vi "Calc Calculated Values 2.vi"(8 "error in":errorcluster, 10 "RT - Analysis Data in":T4={"Accel Sensistivity"=[0.0, 0.0, 0.0], "Cutoff Frequncies"=[{"LP Passband"=0.0, "HP Stopband"=0.0, "LP Stopband"=0.0, "HP Passband"=0.0}, {"LP Passband"=0.0, "HP Stopband"=0.0, "LP Stopband"=0.0, "HP Passband"=0.0}, {"LP Passband"=0.0, "HP Stopband"=0.0, "LP Stopband"=0.0, "HP Passband"=0.0}], "APU Setup File"={"Sensor Info"=[], "CMM Table 106"=[], "CMM Table 106B "=[], "Accel Config"=[], "Report Sheet 1"=[], "Report Sheet 2"=[], "Report Sheet 3"=[]}, "RepairLevel"=""} {"Cutoff Frequncies"."HP Passband" min=1.0 step=1.0 format="%#.4f"; "Cutoff Frequncies"."LP Stopband" min=1.0 step=1.0 format="%#.4f"; "Cutoff Frequncies"."HP Stopband" min=1.0 step=1.0 format="%#.4f"; "Cutoff Frequncies"."LP Passband" min=1.0 step=1.0 format="%#.4f"}, 11 "All Data":T1 caption="All Data Cluster") -> (0 "error out":errorcluster, 3 "Calculated Values out":T3)   [LabVIEW 2018, in "RT - Analysis.lvlib"]
doc: "Performs all calculations to get the calculated values. Default output for a calculated value without an assigned calculation is NaN."
uses:
  RT - Analysis.lvlib
  Top Level/Shared Controls/Calculated Data.ctl
  <userlib>/_OpenG.lib/array/array.llb/Reorder 1D Array2 (DBL)__ogtk.vi
  Private Controls/RT-Analysis Data.ctl
  Modules/Testing UI 3/Private Controls/Cutoff Frequency.ctl
  Modules/Testing UI 3/Testing UI 3.lvlib
  Top Level/Shared Controls/APU Setup File.ctl
  Top Level/Shared Controls/Acq Data.ctl
  Top Level/Shared Controls/All Data Cluster.ctl
panel:
  # "Highpass Cutoff Frequency"
  # "Lowpass Cutoff Frequency"
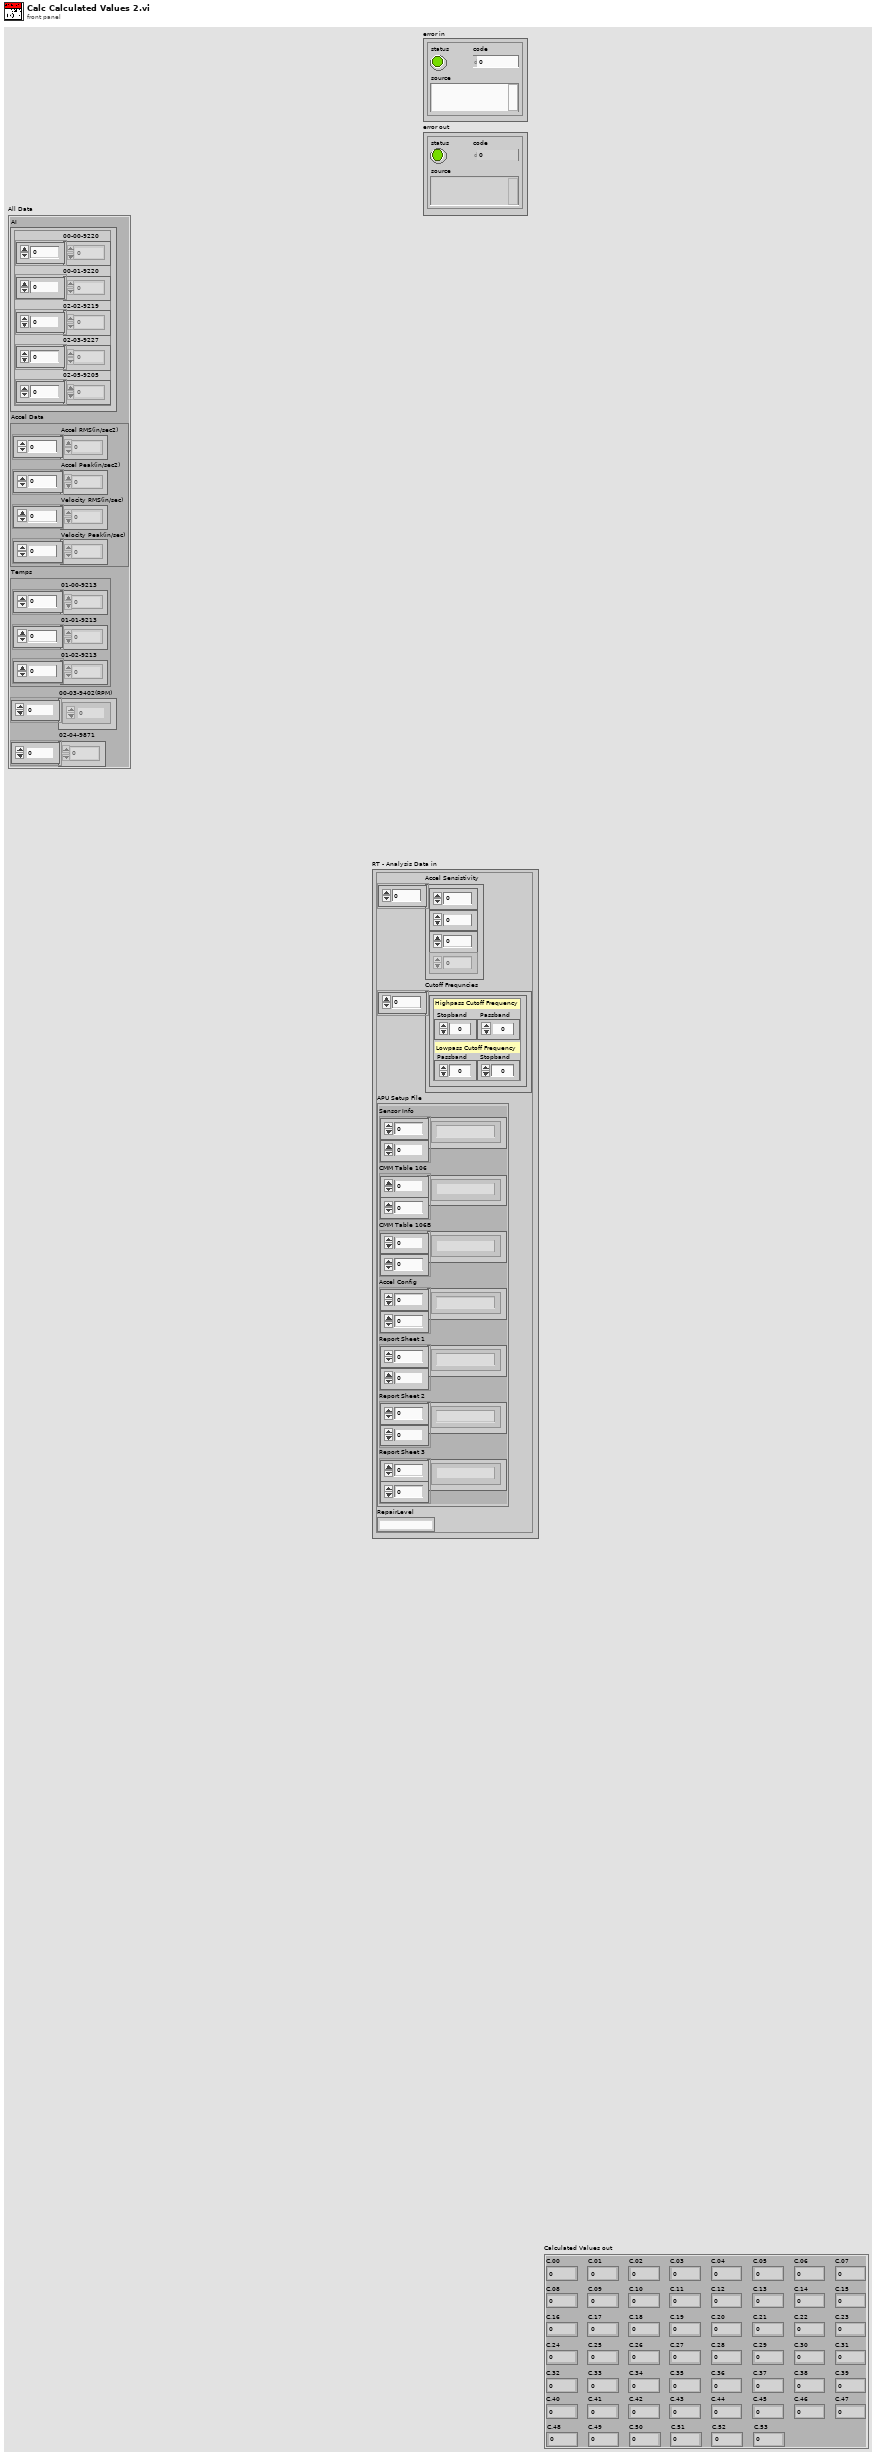
[diagram p1: front panel]
types:
  T1 = typedef "All Data Cluster.ctl" = cluster{"AI":T2, "Accel Data":cluster{"Accel RMS(in/sec2)":dbl[], "Accel Peak(in/sec2)":dbl[], "Velocity RMS(in/sec)":dbl[], "Velocity Peak(in/sec)":dbl[]}, "Temps":cluster{"01-00-9213":dbl[], "01-01-9213":dbl[], "01-02-9213":dbl[]}, "00-03-9402(RPM)":dbl[], "02-04-9871":dbl[]}
  T2 = typedef "Acq Data.ctl" = cluster{"00-00-9220":dbl[], "00-01-9220":dbl[], "02-02-9219":dbl[], "02-03-9227":dbl[], "02-05-9205":dbl[]}
  T3 = typedef "Calculated Data.ctl" = cluster{"C.00":dbl, "C.01":dbl, "C.02":dbl, "C.03":dbl, "C.04":dbl, "C.05":dbl, "C.06":dbl, "C.07":dbl, "C.08":dbl, "C.09":dbl, "C.10":dbl, "C.11":dbl, "C.12":dbl, "C.13":dbl, "C.14":dbl, "C.15":dbl, "C.16":dbl, "C.17":dbl, "C.18":dbl, "C.19":dbl, "C.20":dbl, "C.21":dbl, "C.22":dbl, "C.23":dbl, "C.24":dbl, "C.25":dbl, "C.26":dbl, "C.27":dbl, "C.28":dbl, "C.29":dbl, "C.30":dbl, "C.31":dbl, "C.32":dbl, "C.33":dbl, "C.34":dbl, "C.35":dbl, "C.36":dbl, "C.37":dbl, "C.38":dbl, "C.39":dbl, "C.40":dbl, "C.41":dbl, "C.42":dbl, "C.43":dbl, "C.44":dbl, "C.45":dbl, "C.46":dbl, "C.47":dbl, "C.48":dbl, "C.49":dbl, "C.50":dbl, "C.51":dbl, "C.52":dbl, "C.53":dbl}
  T4 = typedef "RT - Analysis.lvlib/RT-Analysis Data.ctl" = cluster{"Accel Sensistivity":dbl[], "Cutoff Frequncies":T5[], "APU Setup File":T6, "RepairLevel":string}
  T5 = typedef "Testing UI 3.lvlib/Cutoff Frequency.ctl" = cluster{"LP Passband":dbl, "HP Stopband":dbl, "LP Stopband":dbl, "HP Passband":dbl}
  T6 = typedef "APU Setup File.ctl" = cluster{"Sensor Info":string[][], "CMM Table 106":string[][], "CMM Table 106B ":string[][], "Accel Config":string[][], "Report Sheet 1":string[][], "Report Sheet 2":string[][], "Report Sheet 3":string[][]}
  T7 = cluster{"Name":string, "Index":i32, "Length":i32}[]
  T8 = cluster{"Name":string, "Index":i32, "Length":i32}
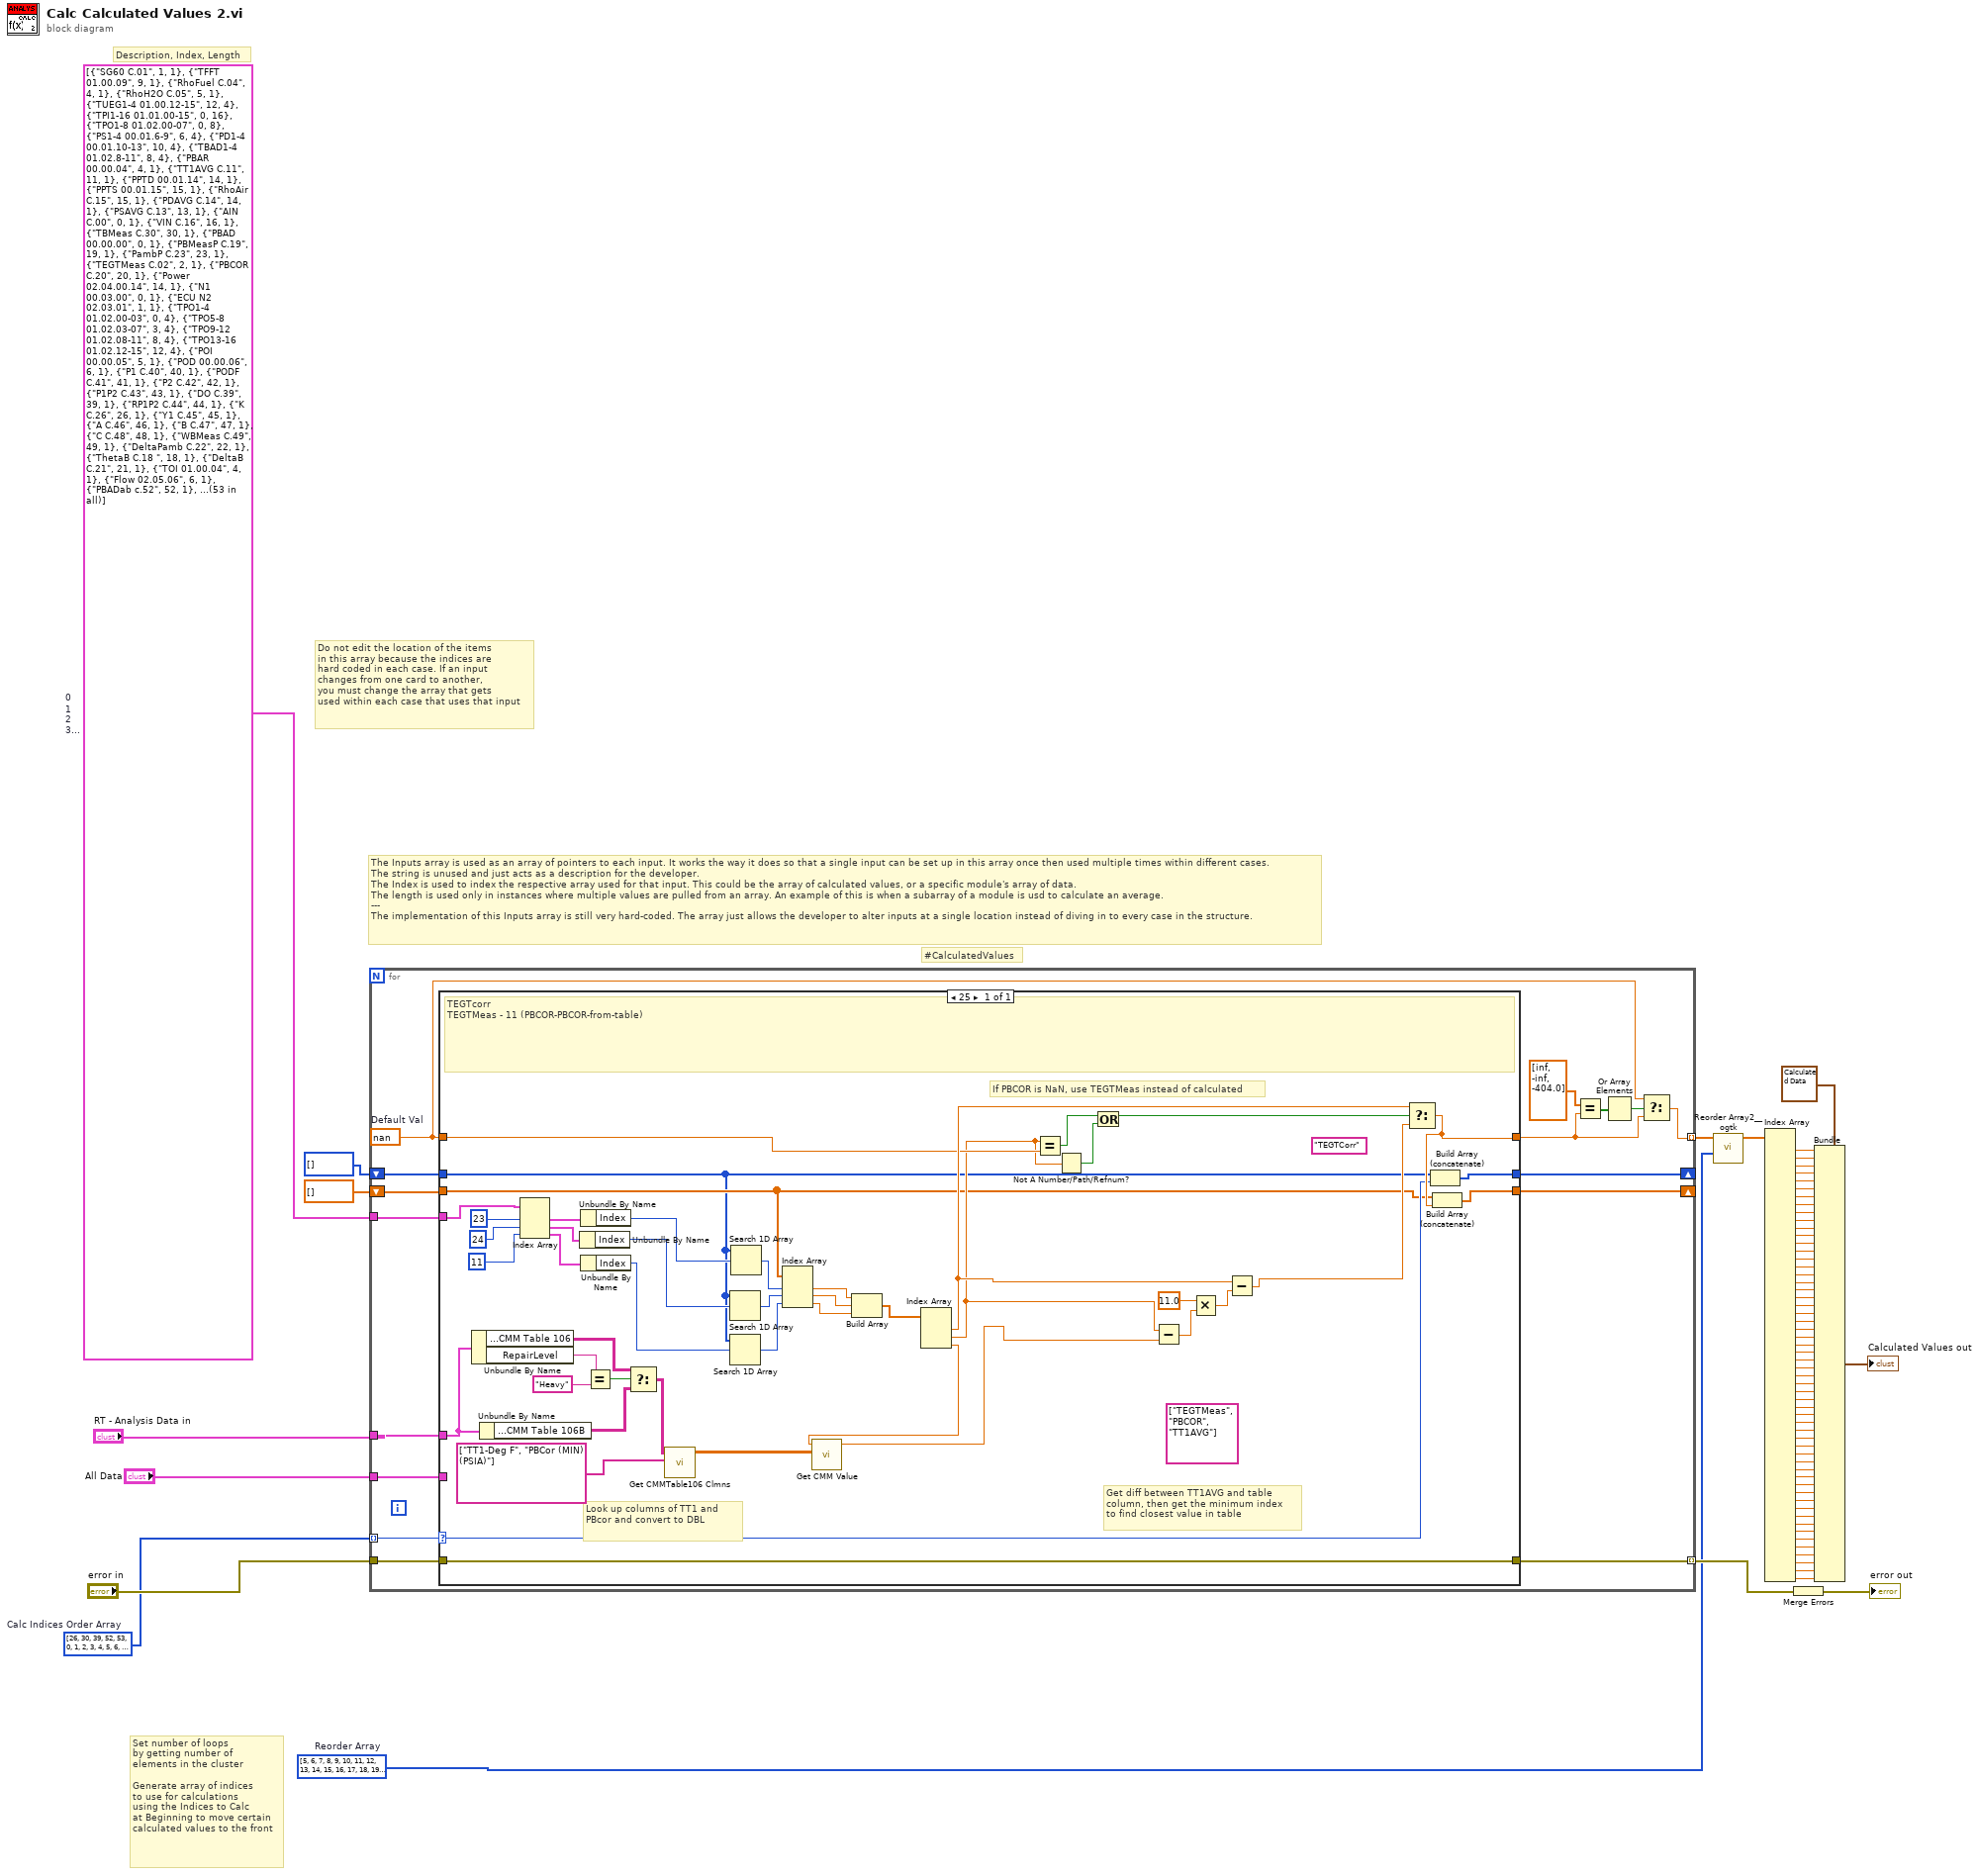
[diagram p0: block diagram]
diagram:
  w2 = i32[] [5, 6, 7, 8, 9, 10, 11, 12, 13, 14, 15, 16, 17, 18, 19, 20, 21, 22, 23, 24, 25, 26, 27, 28, 29, 30, 0, 31, 32, 33, 1, 34, 35, 36, 37, 38, 39, 40, 41, 2, 42, 43, 44, 45, 46, 47, 48, 49, 50, 51, 52, 53, 3, 4, 54, 55]  # Reorder Array
  w3 = i32[] [26, 30, 39, 52, 53, 0, 1, 2, 3, 4, 5, 6, 7, 8, 9, 10, 11, 12, 13, 14, 15, 16, 17, 18, 19, 20, 21, 22, 23, 24, 25, 27, 28, 29, 31, 32, 33, 34, 35, 36, 37, 38, 40, 41, 42, 43, 44, 45, 46, 47, 48, 49, 50, 51, 54, 55]  # Calc Indices Order Array
  w4 = T7 [{"Name"="SG60 C.01", "Index"=1, "Length"=1}, {"Name"="TFFT 01.00.09", "Index"=9, "Length"=1}, {"Name"="RhoFuel C.04", "Index"=4, "Length"=1}, {"Name"="RhoH2O C.05", "Index"=5, "Length"=1}, {"Name"="TUEG1-4 01.00.12-15", "Index"=12, "Length"=4}, {"Name"="TPI1-16 01.01.00-15", "Index"=0, "Length"=16}, {"Name"="TPO1-8 01.02.00-07", "Index"=0, "Length"=8}, {"Name"="PS1-4 00.01.6-9", "Index"=6, "Length"=4}, {"Name"="PD1-4 00.01.10-13", "Index"=10, "Length"=4}, {"Name"="TBAD1-4 01.02.8-11", "Index"=8, "Length"=4}, {"Name"="PBAR 00.00.04", "Index"=4, "Length"=1}, {"Name"="TT1AVG C.11", "Index"=11, "Length"=1}, {"Name"="PPTD 00.01.14", "Index"=14, "Length"=1}, {"Name"="PPTS 00.01.15", "Index"=15, "Length"=1}, {"Name"="RhoAir C.15", "Index"=15, "Length"=1}, {"Name"="PDAVG C.14", "Index"=14, "Length"=1}, {"Name"="PSAVG C.13", "Index"=13, "Length"=1}, {"Name"="AIN C.00", "Index"=0, "Length"=1}, {"Name"="VIN C.16", "Index"=16, "Length"=1}, {"Name"="TBMeas C.30", "Index"=30, "Length"=1}, {"Name"="PBAD 00.00.00", "Index"=0, "Length"=1}, {"Name"="PBMeasP C.19", "Index"=19, "Length"=1}, {"Name"="PambP C.23", "Index"=23, "Length"=1}, {"Name"="TEGTMeas C.02", "Index"=2, "Length"=1}, {"Name"="PBCOR C.20", "Index"=20, "Length"=1}, {"Name"="Power 02.04.00.14", "Index"=14, "Length"=1}, {"Name"="N1 00.03.00", "Index"=0, "Length"=1}, {"Name"="ECU N2 02.03.01", "Index"=1, "Length"=1}, {"Name"="TPO1-4 01.02.00-03", "Index"=0, "Length"=4}, {"Name"="TPO5-8 01.02.03-07", "Index"=3, "Length"=4}, {"Name"="TPO9-12 01.02.08-11", "Index"=8, "Length"=4}, {"Name"="TPO13-16 01.02.12-15", "Index"=12, "Length"=4}, {"Name"="POI 00.00.05", "Index"=5, "Length"=1}, {"Name"="POD 00.00.06", "Index"=6, "Length"=1}, {"Name"="P1 C.40", "Index"=40, "Length"=1}, {"Name"="PODF C.41", "Index"=41, "Length"=1}, {"Name"="P2 C.42", "Index"=42, "Length"=1}, {"Name"="P1P2 C.43", "Index"=43, "Length"=1}, {"Name"="DO C.39", "Index"=39, "Length"=1}, {"Name"="RP1P2 C.44", "Index"=44, "Length"=1}, {"Name"="K C.26", "Index"=26, "Length"=1}, {"Name"="Y1 C.45", "Index"=45, "Length"=1}, {"Name"="A C.46", "Index"=46, "Length"=1}, {"Name"="B C.47", "Index"=47, "Length"=1}, {"Name"="C C.48", "Index"=48, "Length"=1}, {"Name"="WBMeas C.49", "Index"=49, "Length"=1}, {"Name"="DeltaPamb C.22", "Index"=22, "Length"=1}, {"Name"="ThetaB C.18 ", "Index"=18, "Length"=1}, {"Name"="DeltaB C.21", "Index"=21, "Length"=1}, {"Name"="TOI 01.00.04", "Index"=4, "Length"=1}, {"Name"="Flow 02.05.06", "Index"=6, "Length"=1}, {"Name"="PBADab c.52", "Index"=52, "Length"=1}, {"Name"="POIab C.53", "Index"=53, "Length"=1}]  # 0 1 2 3 4 5 6 7 8 9 10 11 12 13 14 15 16 17 18 19 20 21 22 23 24 25 26 27 28 29 30 31 32 33 34 35 36 37 38 39 40 41 42 43 44 45 46 47 48 49 50 51 52
  # "The Inputs array is used as an array of pointers to each input. It works the way it does so that a single input can be set up in this array once then used multiple times within different cases.\nThe string is unused and just acts as a description for the developer.\nThe Index is used to index the respective array used for that input. This could be the array of calculated values, or a specific module's array of data.\nThe length is used only in instances where multiple values are pulled from an array. An example of this is when a subarray of a module is usd to calculate an average.\n---\nThe implementation of this Inputs array is still very hard-coded. The array just allows the developer to alter inputs at a single location instead of diving in to every case in the structure."
  # "Description, Index, Length"
  # "Do not edit the location of the items\nin this array because the indices are\nhard coded in each case. If an input\nchanges from one card to another,\nyou must change the array that gets\nused within each case that uses that input"
  # "#CalculatedValues"
  # "Set number of loops\nby getting number of\nelements in the cluster\n\nGenerate array of indices\nto use for calculations\nusing the Indices to Calc\nat Beginning to move certain\ncalculated values to the front"
  n1 = for {
    tunnel: [w78] -> w8 mode=indexing
    tunnel: [w86] -> w22 mode=indexing
    tunnel: "error in" -> [w85]
    tunnel: "RT - Analysis Data in" -> [w84]
    tunnel: w3 -> [w77] mode=indexing
    shift-right: [w76] -> _
    shift-left: i32[] [] -> [w75]
    shift-right: [w74] -> _
    shift-left: dbl[] [] -> [w73]
    tunnel: w4 -> [w72]
    tunnel: "All Data" -> [w71]
    w80 = nan  # Default Val
    n2 = case shown="25" w77 {
      selector: w77 -> [w117]
      tunnel: w75 -> [w97]
      tunnel: w73 -> [w104]
      tunnel: [w124] -> w79
      tunnel: w80 -> [w122]
      tunnel: [w116] -> w86
      tunnel: w85 -> [w116]
      tunnel: [w131] -> w76
      tunnel: [w130] -> w74
      tunnel: w84 -> [w92]
      tunnel: w72 -> [w109]
      tunnel: w71 -> [_]
      frame 25 {
        (unwired) string[] ["TEGTMeas", "PBCOR", "TT1AVG"]
        (unwired) "TEGTCorr" ("Param")
        # "If PBCOR is NaN, use TEGTMeas instead of calculated"
        # "Get diff between TT1AVG and table\ncolumn, then get the minimum index\nto find closest value in table"
        # "Look up columns of TT1 and PBcor and convert to DBL"
        # "TEGTcorr\nTEGTMeas - 11 (PBCOR-PBCOR-from-table)"
        n3 = Unbundle By Name(w92) -> ("APU Setup File.CMM Table 106"=w96:string[][], "RepairLevel"=w94:string)
        n4 = Unbundle By Name(w92) -> ("APU Setup File.CMM Table 106B"=w91:string[][])
        n5 = Index Array(array=w109, index #1=23 ("index"), index #2=24 ("index"), index #3=11 ("index")) -> (element #1=w115:T8, element #2=w114:T8, element #3=w110:T8)
        n6 = Unbundle By Name(w114) -> ("Index"=w99:i32)
        n7 = Unbundle By Name(w115) -> ("Index"=w100:i32)
        n8 = Unbundle By Name(w110) -> ("Index"=w98:i32)
        n9 = Equal?(x=w94, y="Heavy") -> (x = y?=w95:bool)
        n10 = Select(t=w96, s=w95, f=w91) -> (s? t:f=w90:string[][])
        n11 = call "Get CMMTable106 Clmns.vi"("Column Titles"=string[] ["TT1-Deg F", "PBCor (MIN) (PSIA)"], "[[CMM Table 106]]"=w90) -> ("Columns out"=w128:dbl[][])  [unwired: 9 in]
        n12 = Search 1D Array(1D array=w97, element=w99) -> (index of element=w106:i32)  [unwired: 1 in]
        n13 = Search 1D Array(1D array=w97, element=w98) -> (index of element=w103:i32)  [unwired: 1 in]
        n14 = Search 1D Array(1D array=w97, element=w100) -> (index of element=w108:i32)  [unwired: 1 in]
        n15 = Index Array(array=w104, index #1=w108, index #2=w106, index #3=w103) -> (element #1=w107:dbl, element #2=w105:dbl, element #3=w102:dbl)
        n16 = Build Array(w107, w105, w102) -> (w101:dbl[])
        n17 = Index Array(array=w101) -> (element #1=w123:dbl, element #2=w119:dbl, element #3=w126:dbl)  [unwired: 3 in]
        n18 = call "Get CMM Value.vi"("CMM Table"=w128, "TT1-Deg F C.11"=w126) -> ("Value Out"=w127:dbl)  [unwired: 9 in]
        n19 = Equal?(x=w119, y=w122) -> (x = y?=w121:bool)
        n20 = Not A Number/Path/Refnum?(number/path/refnum=w119) -> (NaN/Path/Refnum?=w118:bool)
        n21 = Or(x=w121, y=w118) -> (x .or. y?=w120:bool)
        n22 = Subtract(x=w119, y=w127) -> (x-y=w89:dbl)
        n23 = Multiply(x=11.0, y=w89) -> (x*y=w87:dbl)
        n24 = Subtract(x=w123, y=w87) -> (x-y=w125:dbl)
        n25 = Select(t=w123, s=w120, f=w125) -> (s? t:f=w124:dbl)
        n26 = Build Array (concatenate)(w97, w117) -> (w131:i32[])
        n27 = Build Array (concatenate)(w104, w124) -> (w130:dbl[])
      }
    }
    n28 = Equal?(x=dbl[] [inf, -inf, -404.0], y=w79) -> (x = y?=w82:bool[])
    n29 = Or Array Elements(Boolean array=w82) -> (logical OR=w81:bool)
    n30 = Select(t=w80, s=w81, f=w79) -> (s? t:f=w78:dbl)
  }
  n31 = call-poly <userlib>:"Reorder Array2__ogtk.vi"("indices"=w2, "array"=w8) -> ("reordered array"=w7:dbl[])  [unwired: 9 in]
  n32 = Index Array(array=w7) -> (element #1=w70:dbl, element #2=w69:dbl, element #3=w68:dbl, element #4=w67:dbl, element #5=w66:dbl, element #6=w65:dbl, element #7=w64:dbl, element #8=w63:dbl, element #9=w62:dbl, element #10=w61:dbl, element #11=w60:dbl, element #12=w59:dbl, element #13=w58:dbl, element #14=w57:dbl, element #15=w56:dbl, element #16=w55:dbl, element #17=w54:dbl, element #18=w53:dbl, element #19=w52:dbl, element #20=w51:dbl, element #21=w50:dbl, element #22=w49:dbl, element #23=w48:dbl, element #24=w47:dbl, element #25=w46:dbl, element #26=w45:dbl, element #27=w44:dbl, element #28=w43:dbl, element #29=w42:dbl, element #30=w41:dbl, element #31=w40:dbl, element #32=w39:dbl, element #33=w38:dbl, element #34=w37:dbl, element #35=w36:dbl, element #36=w35:dbl, element #37=w34:dbl, element #38=w33:dbl, element #39=w32:dbl, element #40=w31:dbl, element #41=w30:dbl, element #42=w29:dbl, element #43=w28:dbl, element #44=w27:dbl, element #45=w26:dbl, element #46=w25:dbl, element #47=w24:dbl, element #48=w23:dbl, element #49=w17:dbl, element #50=w16:dbl, element #51=w15:dbl, element #52=w14:dbl, element #53=w13:dbl, element #54=w12:dbl, element #55=w11:dbl, element #56=w10:dbl)  [unwired: 56 in]
  n33 = Merge Errors(w22) -> (→"error out":errorcluster)
  n34 = Bundle(cluster=T3 {"C.00"=0.0, "C.01"=0.0, "C.02"=0.0, "C.03"=0.0, "C.04"=0.0, "C.05"=0.0, "C.06"=0.0, "C.07"=0.0, "C.08"=0.0, "C.09"=0.0, "C.10"=0.0, "C.11"=0.0, "C.12"=0.0, "C.13"=0.0, "C.14"=0.0, "C.15"=0.0, "C.16"=0.0, "C.17"=0.0, "C.18"=0.0, "C.19"=0.0, "C.20"=0.0, "C.21"=0.0, "C.22"=0.0, "C.23"=0.0, "C.24"=0.0, "C.25"=0.0, "C.26"=0.0, "C.27"=0.0, "C.28"=0.0, "C.29"=0.0, "C.30"=0.0, "C.31"=0.0, "C.32"=0.0, "C.33"=0.0, "C.34"=0.0, "C.35"=0.0, "C.36"=0.0, "C.37"=0.0, "C.38"=0.0, "C.39"=0.0, "C.40"=0.0, "C.41"=0.0, "C.42"=0.0, "C.43"=0.0, "C.44"=0.0, "C.45"=0.0, "C.46"=0.0, "C.47"=0.0, "C.48"=0.0, "C.49"=0.0, "C.50"=0.0, "C.51"=0.0, "C.52"=0.0, "C.53"=0.0} ("Calculated Values out"), w70, w69, w68, w67, w66, w65, w64, w63, w62, w61, w60, w59, w58, w57, w56, w55, w54, w53, w52, w51, w50, w49, w48, w47, w46, w45, w44, w43, w42, w41, w40, w39, w38, w37, w36, w35, w34, w33, w32, w31, w30, w29, w28, w27, w26, w25, w24, w23, w17, w16, w15, w14, w13, w12, w11, w10) -> (→"Calculated Values out":T3)
